vi "Get Descriptor Byte.vi"(8 "Error In":errorcluster, 11 "Data Set":T1=enum."NAV") -> (0 "Error Out":errorcluster, 3 "Desciptor Byte":u8 format="%x")   [LabVIEW 2011]
doc: "The three data sets represent the three types of data that the 3DM-GX3-45 is capable of producing: “AHRS” (Attitude and Heading Reference System) data, “GPS” (Global Positioning Sensor) data, and “NAV” (Navigation) data.\n\nThe VI selects the correct Descriptor Byte for the desired data set"
uses:
  Controls/Desciptor Set Byte.ctl
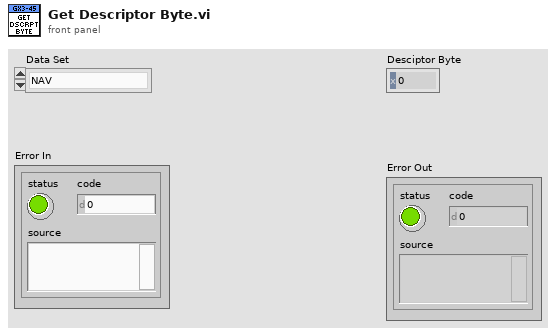
[diagram p1: front panel]
types:
  T1 = typedef "Desciptor Set Byte.ctl" = enum16{"Base Command Set", "3DM Command Set", "Navigation Filter Command Set", "System Command Set", "AHRS", "GPS", "NAV"}
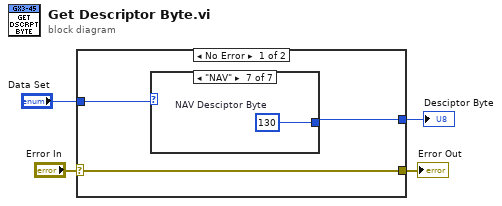
[diagram p0: block diagram]
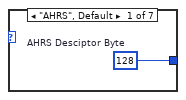
[diagram p2: hidden frame]
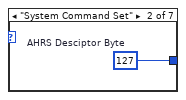
[diagram p3: hidden frame]
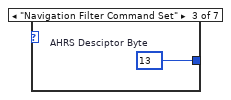
[diagram p4: hidden frame]
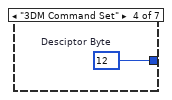
[diagram p5: hidden frame]
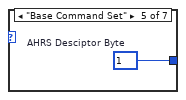
[diagram p6: hidden frame]
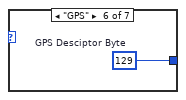
[diagram p7: hidden frame]
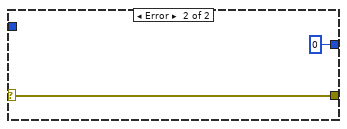
[diagram p8: hidden frame]
diagram:
  n1 = case shown="No Error" "Error In" {
    selector: "Error In" -> [w7 w16]
    tunnel: [w7 w16] -> w3
    tunnel: "Data Set" -> [w6 _]
    tunnel: [w5 u8 0 ("NAV Desciptor Byte")] -> w1
    frame No Error {
      n2 = case shown="\"NAV\"" w6 {
        tunnel: [w8 w9 w10 w11 w12 w13 w14] -> w5
        frame "AHRS", Default {
          w8 = u8 128  # AHRS Desciptor Byte
        }
        frame "System Command Set" {
          w9 = u8 127  # AHRS Desciptor Byte
        }
        frame "Navigation Filter Command Set" {
          w10 = u8 13  # AHRS Desciptor Byte
        }
        frame "3DM Command Set" {
          w11 = u8 12  # Desciptor Byte
        }
        frame "Base Command Set" {
          w12 = u8 1  # AHRS Desciptor Byte
        }
        frame "GPS" {
          w13 = u8 129  # GPS Desciptor Byte
        }
        frame "NAV" {
          w14 = u8 130  # NAV Desciptor Byte
        }
      }
    }
    frame Error {
    }
  }
  "Error Out" <- w3
  "Desciptor Byte" <- w1
